vi "ReadPersistentConfiguration.vi"(8 "ErrorIn":errorcluster, 10 "DataIn":variant, 11 "ObjectIn":refnum<class "YAFTAF.lvclass">) -> (0 "ErrorOut":errorcluster, 2 "DataOut":variant, 3 "ObjectOut":refnum<class "YAFTAF.lvclass">)   [LabVIEW 2021, in "YAFTAF.lvclass"]
uses:
  YAFTAF.lvclass
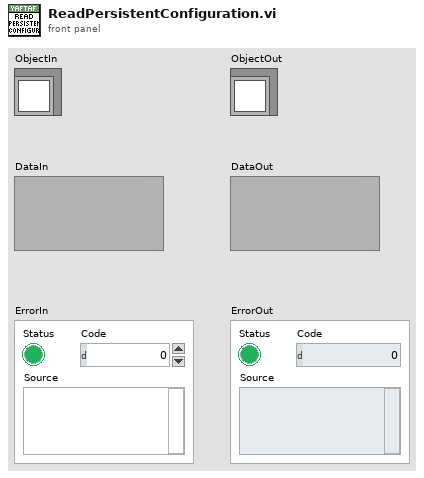
[diagram p1: front panel]
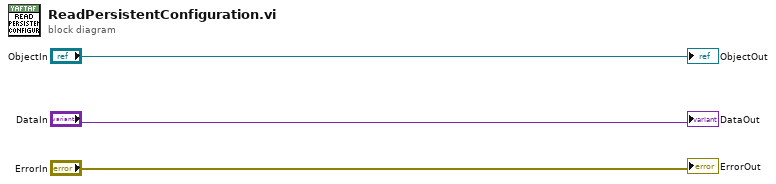
[diagram p0: block diagram]
diagram:
  "ErrorOut" <- "ErrorIn"
  "ObjectOut" <- "ObjectIn"
  "DataOut" <- "DataIn"
